vi "encoderData.vi"() -> ()   [LabVIEW 2014]
panel:
  in  "LiftVelocity":dbl
  in  "LiftDistance":dbl
  in  "AverageDistance":dbl
  in  "AverageStrafeDistance":dbl
  in  "BackDistance":dbl
  in  "BackVelocity":dbl
  in  "FrontDistance":dbl
  in  "FrontVelocity":dbl
  in  "LeftDistance":dbl
  in  "LeftVelocity":dbl
  in  "RightDistance":dbl
  in  "RightVelocity":dbl
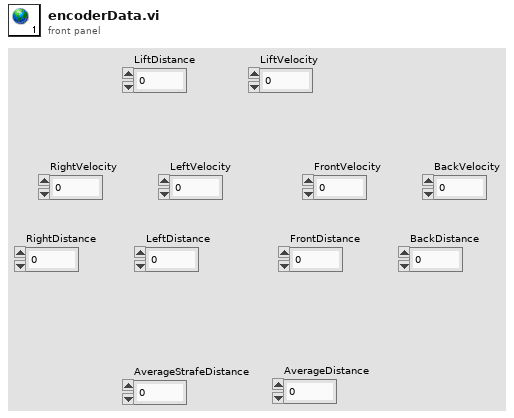
[diagram p1: front panel]
diagram:
